vi "crio_RT_LAC.vi"() -> ()   [LabVIEW 2019]
uses:
  <vilib>/FPGAPlugInAG/cRIO-9074/niLvFpga_Open_cRIO-9074.vi
  <vilib>/rvi/interface/common/dynamic/niFpgaDynamicAddResources.vi
  <vilib>/FPGAPlugInAG/Dynamic/niLvFpga_Run_Dynamic.vi
  <vilib>/Utility/error.llb/Error Cluster From Error Code.vi
  <vilib>/rvi/errors/niLvFpgaAdjustHostInterfaceError.vi
  <vilib>/FPGAPlugInAG/Dynamic/niLvFpga_Close_Dynamic.vi
  <vilib>/rvi/interface/nirviOpenFPGA/nirviOpenFPGA.xnode
  FPGA Bitfiles/gpass2_FPGATarget2_crioFPGALAC2_Q4l8kPWlMdE.lvbitx
  crio_FPGA_LAC.vi
  <vilib>/rvi/interface/nirviMethod/nirviMethod.xnode
  <vilib>/rvi/interface/nirviReadWriteControl/nirviReadWriteControl.xnode
  <vilib>/rvi/interface/nirviCloseFPGA/nirviCloseFPGA.xnode
  NiFpgaLv.dll
  <vilib>/rvi/interface/Simulation/niFpgaSimulationCallBeginRW.vi
panel:
  in  "Select":enum16{"User defined", "Sine"}(ring)
  in  "Angle (deg)":dbl(slide) scale=-90.0..90.0
  in  "Stop":bool
  out "pulse width (us)":i32
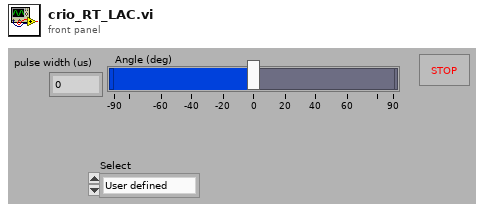
[diagram p1: front panel]
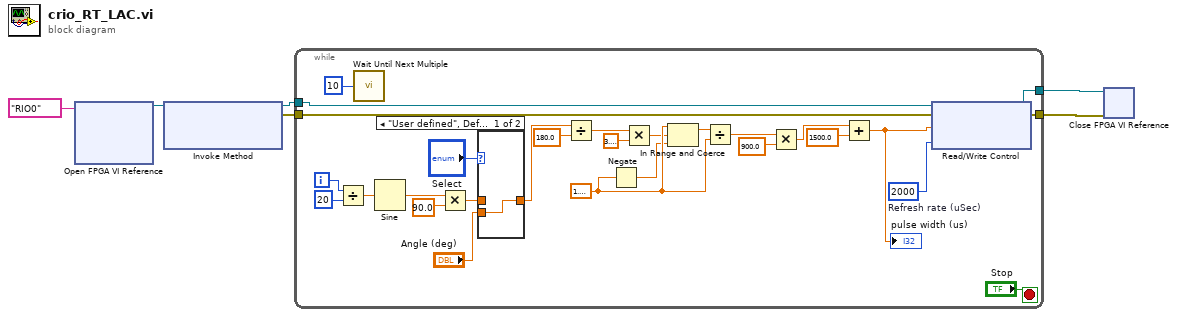
[diagram p0: block diagram]
diagram:
  n1 = xnode "Open FPGA VI Reference"("resource name"=tag "RIO0") -> ("FPGA VI Reference Out"=w2:refnum<k20>)  [unwired: 1 in, 1 out]
  n2 = xnode "Invoke Method"("FPGA VI Reference In"=w2) -> ("FPGA VI Reference Out"=w6:refnum<k20>, "error out"=w5:errorcluster)  [unwired: 2 in]
  n3 = while {
    tunnel: w6 -> [w34]
    tunnel: w5 -> [w33]
    tunnel: [w23] -> w4
    tunnel: [w22] -> w3
    i -> [w13]
    stop <- "Stop" stop-if-true
    w21 = u32 2000  # Refresh rate (uSec)
    w28 = 1.5707963267948966
    n4 = Divide(x=w13, y=20) -> (x/y=w12:dbl)
    n5 = call "Wait Until Next Multiple"("Count(mSec)"=u32 10) -> ()  [unwired: 1 out]
    n6 = Sine(x=w12) -> (sin(x)=w15:dbl)
    n7 = Multiply(x=w15, y=90.0) -> (x*y=w10:dbl)
    n8 = case shown="\"User defined\", Default" "Select" {
      tunnel: w10 -> [_ w36]
      tunnel: "Angle (deg)" -> [w35 _]
      tunnel: [w35 w36] -> w8
      frame "User defined", Default {
      }
      frame "Sine" {
      }
    }
    n9 = Divide(x=w8, y=180.0) -> (x/y=w19:dbl)
    n10 = Negate(x=w28) -> (-x=w26:dbl)
    n11 = Multiply(x=w19, y=3.141592653589793) -> (x*y=w18:dbl)
    n12 = In Range and Coerce(upper limit=w28, x=w18, lower limit=w26) -> (coerced(x)=w27:dbl)  [unwired: 1 out]
    n13 = Divide(x=w27, y=w28) -> (x/y=w29:dbl)
    n14 = Multiply(x=w29, y=900.0) -> (x*y=w31:dbl)
    n15 = Add(x=w31, y=1500.0) -> (x+y=w25:dbl)
    "pulse width (us)" <- w25
    n16 = xnode "Read/Write Control"("FPGA VI Reference In"=w34, "error in"=w33, "Servo wait time"=w25, "Count(uSec)"=w21) -> ("FPGA VI Reference Out"=w23:refnum<k20>, "error out"=w22:errorcluster)
  }
  n17 = xnode "Close FPGA VI Reference"("FPGA VI Reference In"=w4, "error in"=w3) -> ()  [unwired: 1 out]
